vi "ConvertTriggerEventsToEventList.vi"(11 "Trigger Events":enum16{"Source", "Delay", "Sense", "None"}[](array[ring])) -> (3 "Event List":string)   [LabVIEW 8.6, in "Keithley-6482-Visa.lvlib"]
uses:
  Keithley-6482-Visa.lvlib
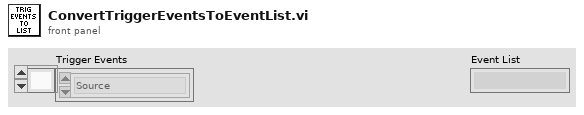
[diagram p1: front panel]
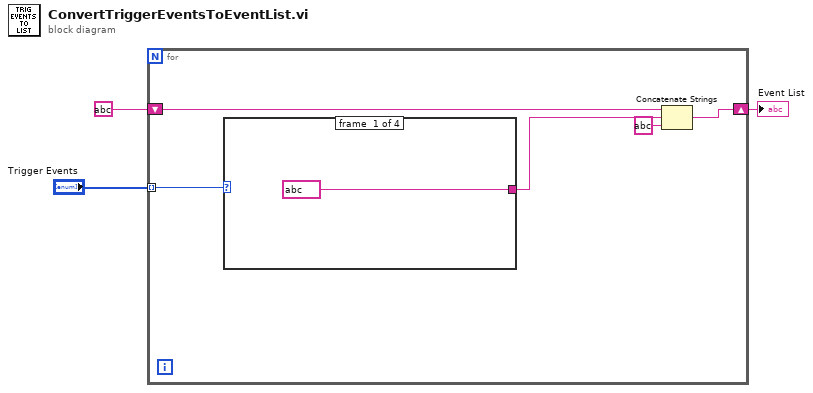
[diagram p0: block diagram]
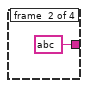
[diagram p2: hidden frame]
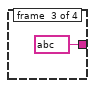
[diagram p3: hidden frame]
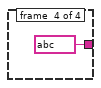
[diagram p4: hidden frame]
diagram:
  n1 = for {
    tunnel: "Trigger Events" -> [w6] mode=indexing
    shift-right: [w7] -> w1
    shift-left: string ? -> [w8]
    n2 = case shown="\"None\"" w6 {
      tunnel: [string ? string ? string ? string ?] -> w5
      frame #0 {
      }
      frame #1 {
      }
      frame #2 {
      }
      frame #3 {
      }
    }
    n3 = Concatenate Strings(w8, w5, string ? ("string")) -> (w7:string)
  }
  "Event List" <- w1
